vi "SerialOpen.vi"(1 "串口配置":T1={"VISA资源名称"="COM1", "波特率"=9600, "数据位"=8, "校验"=enum."None", "停止位"=enum."2.0"} {"数据位" min=5 max=8 step=1; "波特率" items=["75"=75, "110"=110, "134"=134, "150"=150, "300"=300, "600"=600, "1200"=1200, "1800"=1800, "2400"=2400, "4800"=4800, "7200"=7200, "9600"=9600, "14400"=14400, "19200"=19200, "28800"=28800, "38400"=38400, "56000"=56000, "57600"=57600, "115200"=115200, "128000"=128000, "230400"=230400]}) -> (0 "VISA resource name out":refnum<visa-resource-name>)   [LabVIEW 2019]
uses:
  <vilib>/Instr/_visa.llb/VISA Configure Serial Port (Instr).vi
panel:
  # "串口号："
  # "停止位："
  # "校验位"
  # "数据位："
  # "波特率："
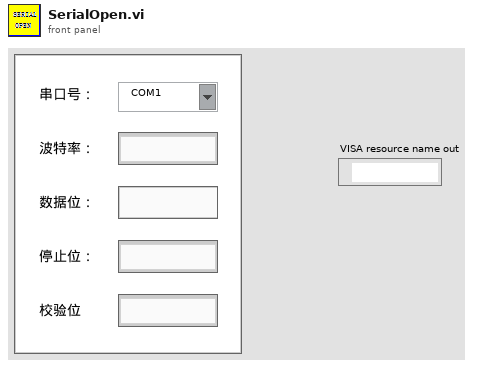
[diagram p1: front panel]
types:
  T1 = cluster{"VISA资源名称":refnum<visa-resource-name>, "波特率":u32, "数据位":u16, "校验":enum16{"None", "Odd", "Even", "Mark", "Space"}, "停止位":enum16{"1.0", "1.5", "2.0"}}
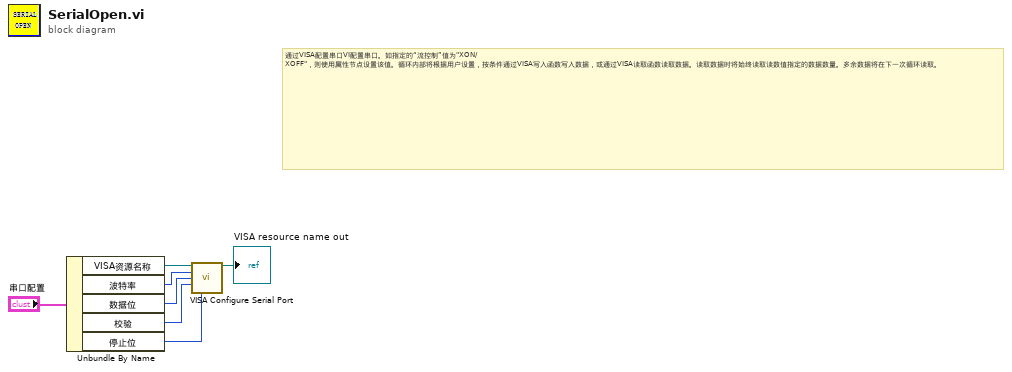
[diagram p0: block diagram]
diagram:
  # "通过VISA配置串口VI配置串口。如指定的“流控制”值为\"XON/XOFF\"，则使用属性节点设置该值。循环内部将根据用户设置，按条件通过VISA写入函数写入数据，或通过VISA读取函数读取数据。读取数据时将始终读取读数值指定的数据数量。多余数据将在下一次循环读取。"
  n1 = Unbundle By Name("串口配置") -> ("VISA资源名称"=w2:refnum<visa-resource-name>, "波特率"=w6:u32, "数据位"=w5:u16, "校验"=w4:enum16{"None", "Odd", "Even", "Mark", "Space"}, "停止位"=w3:enum16{"1.0", "1.5", "2.0"})
  n2 = call-poly "VISA Configure Serial Port"("VISA resource name"=w2, "baud rate (9600)"=w6, "data bits (8)"=w5, "parity (0:none)"=w4, "stop bits (10: 1 bit)"=w3) -> ("VISA resource name out"=→"VISA resource name out":refnum<visa-resource-name>)  [unwired: 5 in, 5 out]
